vi "insertHTBinData.vi"() -> ()   [LabVIEW 2012]
uses:
  <vilib>/addons/database/Connection.llb/Conn ObjectReference.ctl
  <vilib>/addons/database/NI_Database_API.lvlib
panel:
  in  "FileName":string
  out "error out":errorcluster
  out "connection reference out":T1
  in  "error in (no error)":errorcluster
  in  "connection reference":T1
  in  "string":string
  out "concatenated string":string
  in  "input cluster":T2
  out "after substring":string
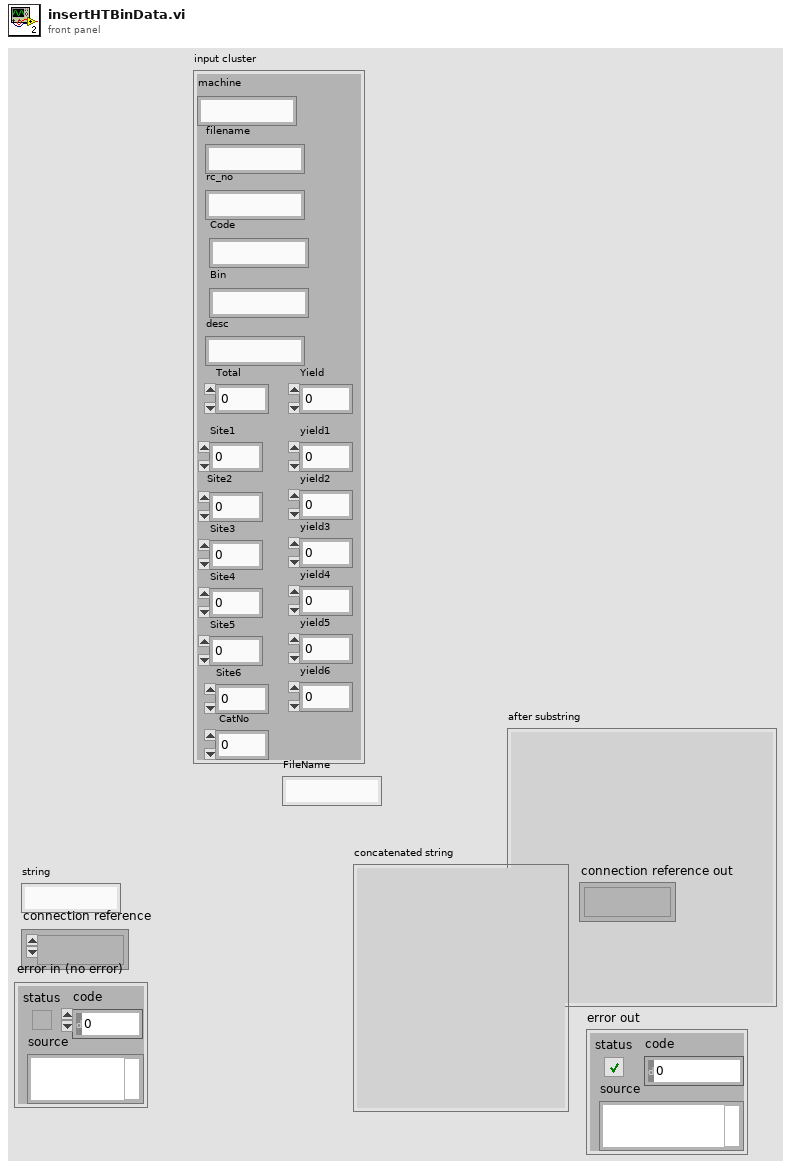
[diagram p1: front panel]
types:
  T1 = typedef "NI_Database_API.lvlib/Conn ObjectReference.ctl" = refnum<k1>
  T2 = cluster{"machine":string, "filename":string, "rc_no":string, "Code":string, "Bin":string, "desc":string, "Total":dbl, "Yield":dbl, "Site1":dbl, "yield1":dbl, "Site2":dbl, "yield2":dbl, "Site3":dbl, "yield3":dbl, "Site4":dbl, "yield4":dbl, "Site5":dbl, "yield5":dbl, "Site6":dbl, "yield6":dbl, " CatNo":dbl}
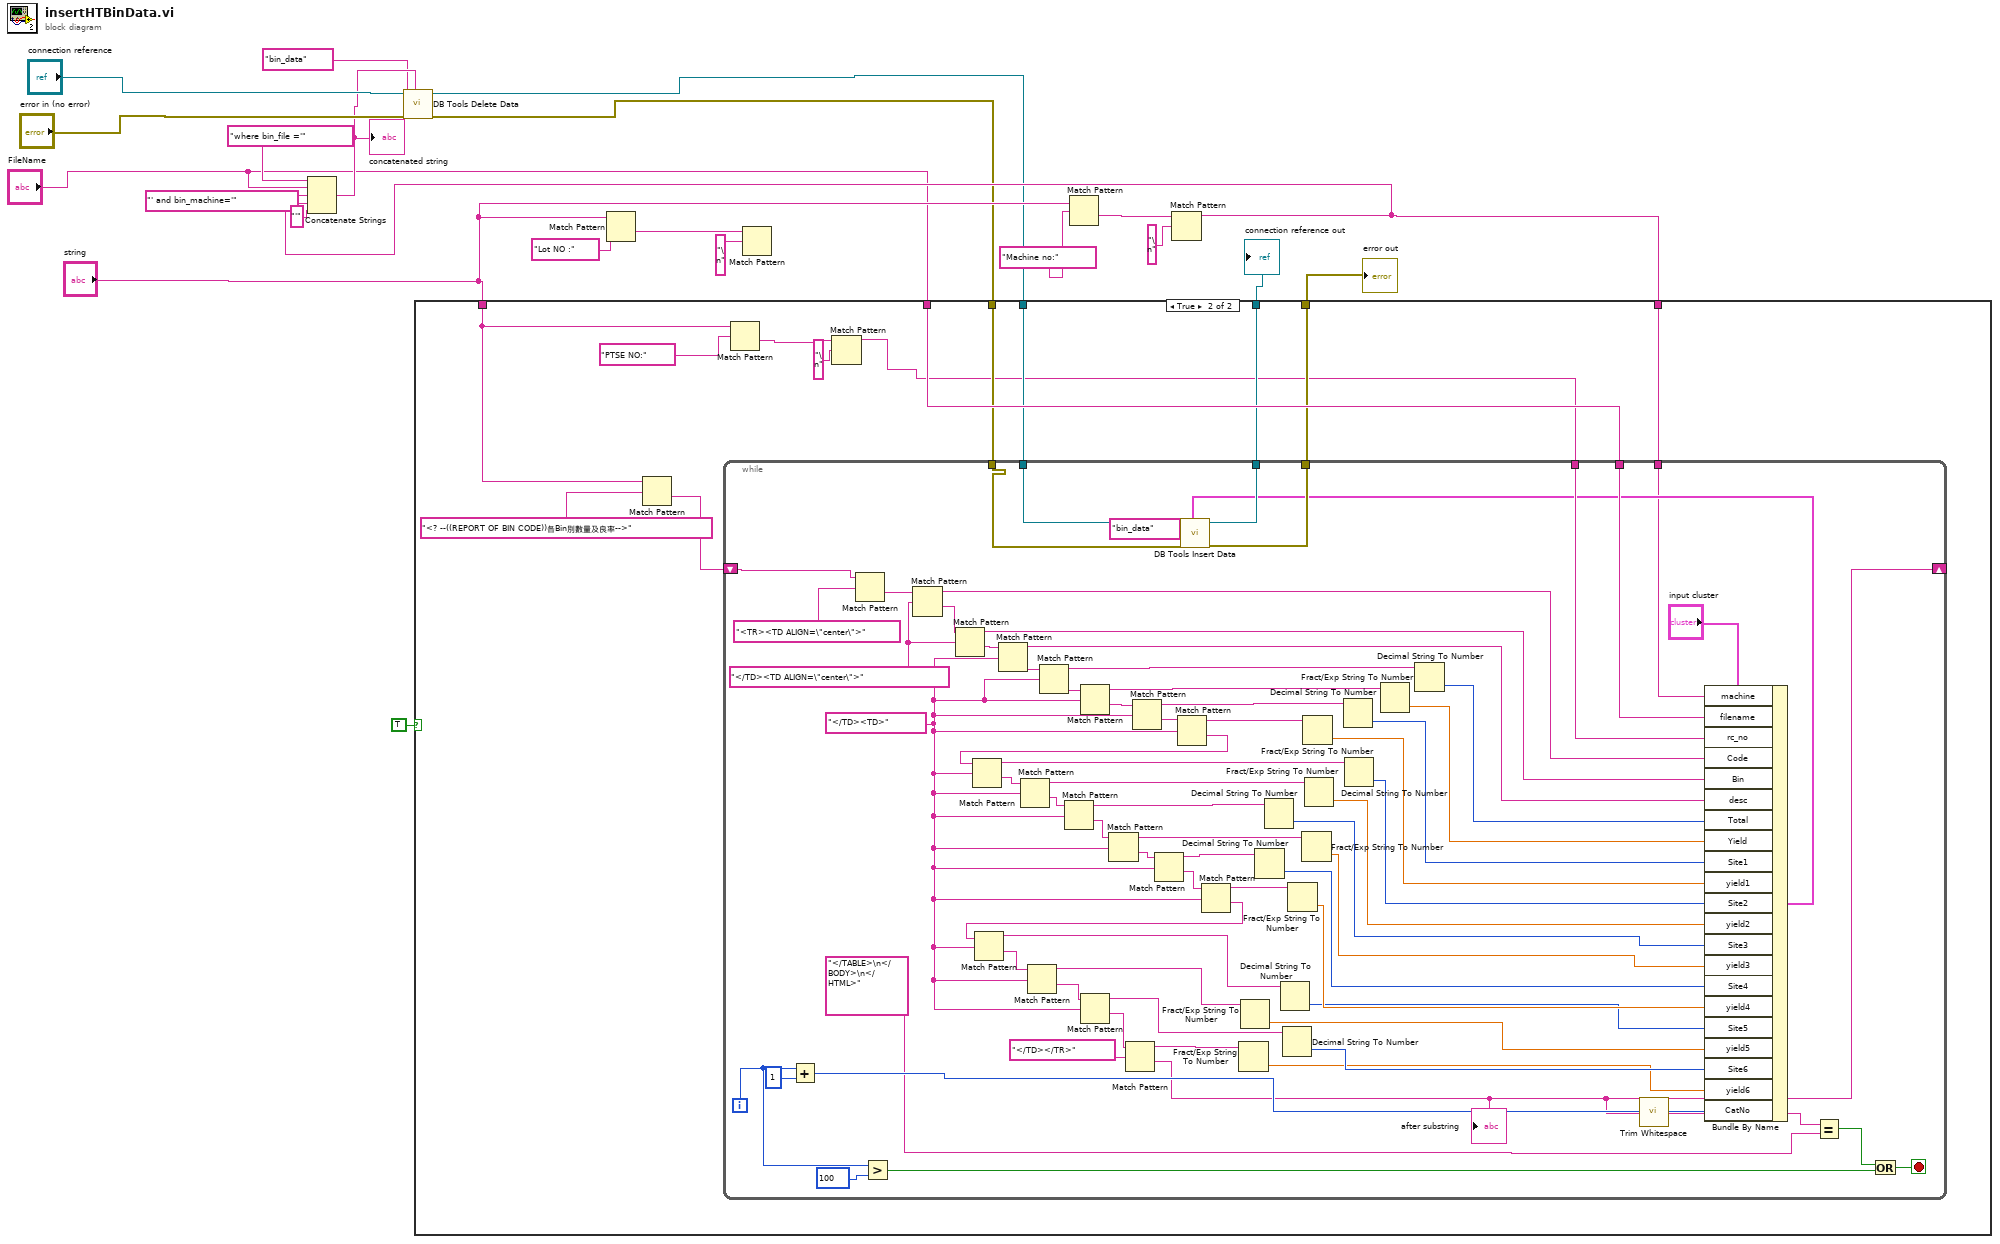
[diagram p0: block diagram]
diagram:
  n1 = Match Pattern(string="string", regular expression="Lot NO :") -> (after substring=w18:string)  [unwired: 1 in, 3 out]
  n2 = Match Pattern(string=w18, regular expression="\n") -> ()  [unwired: 1 in, 4 out]
  n3 = Match Pattern(string="string", regular expression="Machine no:") -> (after substring=w10:string)  [unwired: 1 in, 3 out]
  n4 = Match Pattern(string=w10, regular expression="\n") -> (before substring=w7:string)  [unwired: 1 in, 3 out]
  n5 = Concatenate Strings("where bin_file ='" ("SQL query"), "FileName", "' and bin_machine='" ("string"), w7, "'" ("string")) -> (w5:string)
  "concatenated string" <- w5
  n6 = call <vilib>:"DB Tools Delete Data.vi"("condition"=w5, "error in (no error)"="error in (no error)", "table"="bin_data", "connection reference"="connection reference") -> ("error out"=w2:errorcluster, "connection reference out"=w3:T1)  [unwired: 6 in]
  n7 = case shown="True" TRUE {
    tunnel: "string" -> [_ w33]
    tunnel: "FileName" -> [_ w31]
    tunnel: w3 -> [w23 w30]
    tunnel: [w23 w29] -> w21
    tunnel: [w22 w28] -> w20
    tunnel: w2 -> [w22 w27]
    tunnel: w7 -> [_ w26]
    frame False {
    }
    frame True {
      n8 = Match Pattern(string=w33, regular expression="<? --((REPORT OF BIN CODE))各Bin別數量及良率-->") -> (after substring=w32:string)  [unwired: 1 in, 3 out]
      n9 = Match Pattern(string=w33, regular expression="PTSE NO:") -> (after substring=w35:string)  [unwired: 1 in, 3 out]
      n10 = Match Pattern(string=w35, regular expression="\n") -> (before substring=w25:string)  [unwired: 1 in, 3 out]
      n11 = while {
        shift-right: [w43] -> _
        shift-left: w32 -> [w89]
        tunnel: w31 -> [w86]
        tunnel: w25 -> [w85]
        tunnel: w30 -> [w52]
        tunnel: [w51] -> w29
        tunnel: [w50] -> w28
        tunnel: w27 -> [w48]
        tunnel: w26 -> [w47]
        i -> [w39]
        stop <- w41 stop-if-true
        w90 = "</TD><TD>" ("regular expression")
        w105 = "</TD><TD ALIGN=\"center\">" ("regular expression")
        n12 = Add(x=w39, y=1) -> (x+y=w45:i32)
        n13 = Match Pattern(string=w89, regular expression="<TR><TD ALIGN=\"center\">") -> (after substring=w108:string)  [unwired: 1 in, 3 out]
        n14 = Greater?(x=w39, y=100) -> (0:w37:bool)
        n15 = Match Pattern(string=w108, regular expression=w105) -> (before substring=w84:string, after substring=w107:string)  [unwired: 1 in, 2 out]
        n16 = Match Pattern(string=w107, regular expression=w105) -> (before substring=w83:string, after substring=w106:string)  [unwired: 1 in, 2 out]
        n17 = Match Pattern(string=w106, regular expression=w90) -> (before substring=w82:string, after substring=w104:string)  [unwired: 1 in, 2 out]
        n18 = Match Pattern(string=w104, regular expression=w90) -> (before substring=w80:string, after substring=w103:string)  [unwired: 1 in, 2 out]
        n19 = Match Pattern(string=w103, regular expression=w90) -> (before substring=w79:string, after substring=w102:string)  [unwired: 1 in, 2 out]
        n20 = Match Pattern(string=w102, regular expression=w90) -> (before substring=w78:string, after substring=w101:string)  [unwired: 1 in, 2 out]
        n21 = Match Pattern(string=w101, regular expression=w90) -> (before substring=w74:string, after substring=w100:string)  [unwired: 1 in, 2 out]
        n22 = Match Pattern(string=w100, regular expression=w90) -> (before substring=w72:string, after substring=w99:string)  [unwired: 1 in, 2 out]
        n23 = Match Pattern(string=w99, regular expression=w90) -> (before substring=w71:string, after substring=w98:string)  [unwired: 1 in, 2 out]
        n24 = Match Pattern(string=w98, regular expression=w90) -> (before substring=w69:string, after substring=w97:string)  [unwired: 1 in, 2 out]
        n25 = Match Pattern(string=w97, regular expression=w90) -> (before substring=w67:string, after substring=w96:string)  [unwired: 1 in, 2 out]
        n26 = Match Pattern(string=w96, regular expression=w90) -> (before substring=w64:string, after substring=w95:string)  [unwired: 1 in, 2 out]
        n27 = Match Pattern(string=w95, regular expression=w90) -> (before substring=w62:string, after substring=w91:string)  [unwired: 1 in, 2 out]
        n28 = Match Pattern(string=w91, regular expression=w90) -> (before substring=w60:string, after substring=w94:string)  [unwired: 1 in, 2 out]
        n29 = Match Pattern(string=w94, regular expression=w90) -> (before substring=w56:string, after substring=w93:string)  [unwired: 1 in, 2 out]
        n30 = Match Pattern(string=w93, regular expression=w90) -> (before substring=w55:string, after substring=w92:string)  [unwired: 1 in, 2 out]
        n31 = Match Pattern(string=w92, regular expression="</TD></TR>") -> (before substring=w54:string, after substring=w43:string)  [unwired: 1 in, 2 out]
        "after substring" <- w43
        n32 = Fract/Exp String To Number(string=w54) -> (number=w57:dbl)  [unwired: 3 in, 1 out]
        n33 = Fract/Exp String To Number(string=w56) -> (number=w59:dbl)  [unwired: 3 in, 1 out]
        n34 = Decimal String To Number(string=w64) -> (number=w66:i32)  [unwired: 2 in, 1 out]
        n35 = Decimal String To Number(string=w69) -> (number=w68:i32)  [unwired: 2 in, 1 out]
        n36 = Decimal String To Number(string=w60) -> (number=w61:i32)  [unwired: 2 in, 1 out]
        n37 = Decimal String To Number(string=w55) -> (number=w58:i32)  [unwired: 2 in, 1 out]
        n38 = Fract/Exp String To Number(string=w62) -> (number=w63:dbl)  [unwired: 3 in, 1 out]
        n39 = Fract/Exp String To Number(string=w67) -> (number=w65:dbl)  [unwired: 3 in, 1 out]
        n40 = Fract/Exp String To Number(string=w74) -> (number=w75:dbl)  [unwired: 3 in, 1 out]
        n41 = Fract/Exp String To Number(string=w71) -> (number=w70:dbl)  [unwired: 3 in, 1 out]
        n42 = Decimal String To Number(string=w78) -> (number=w76:i32)  [unwired: 2 in, 1 out]
        n43 = Decimal String To Number(string=w72) -> (number=w73:i32)  [unwired: 2 in, 1 out]
        n44 = Fract/Exp String To Number(string=w79) -> (number=w77:dbl)  [unwired: 3 in, 1 out]
        n45 = Decimal String To Number(string=w80) -> (number=w81:i32)  [unwired: 2 in, 1 out]
        n46 = call <vilib>:"Trim Whitespace.vi"("string"=w43) -> ("trimmed string"=w42:string)  [unwired: 1 in]
        n47 = Bundle By Name(cluster="input cluster", "machine"=w47, "filename"=w86, "rc_no"=w85, "Code"=w84, "Bin"=w83, "desc"=w82, "Total"=w81, "Yield"=w77, "Site1"=w76, "yield1"=w75, "Site2"=w73, "yield2"=w70, "Site3"=w68, "yield3"=w65, "Site4"=w66, "yield4"=w63, "Site5"=w61, "yield5"=w59, "Site6"=w58, "yield6"=w57, "CatNo"=w45) -> (w49:T2)
        n48 = call <vilib>:"DB Tools Insert Data.vi"("data"=w49, "error in (no error)"=w48, "table"="bin_data", "connection reference"=w52) -> ("error out"=w50:errorcluster, "connection reference out"=w51:T1)  [unwired: 6 in]
        n49 = Equal?(x=w42, y="</TABLE>\n</BODY>\n</HTML>") -> (x = y?=w40:bool)
        n50 = Or(x=w40, y=w37) -> (x .or. y?=w41:bool)
      }
    }
  }
  "connection reference out" <- w21
  "error out" <- w20
